vi "Global_ACT_Data Out.vi"() -> ()   [LabVIEW 2023, in "RingPlacer_ACT.lvlib"]
uses:
  startup.rtexe/RingPlacer_ACT.lvlib
  Cluster_Shooter Status.ctl
  startup.rtexe/Cluster_Speed Sensor Values.ctl
  startup.rtexe/Cluster_Velocity Values.ctl
  startup.rtexe/Cluster_Voltage Values.ctl
  startup.rtexe/Spark MAX Control Type.ctl
  startup.rtexe/Shooter_ACT.lvlib
panel:
  in  "ACT_RingPlacer_Control Mode":T1
  in  "ACT_RingPlacer_Status":T2
  in  "ACT_RingPlacer Motor Value":dbl
  in  "ACT_RingPlacer_CycleTime(S)":dbl
  # "The Names of the Data items in the Global Variable MUST describe who the Single Writer is\nFor Actuator Globals the the naming convention is\n   \nACT_Lib Name_Data Name\n\nExamples:\nACT_Drive_X axis\nACT_Hopper_AgitatorSpeed"
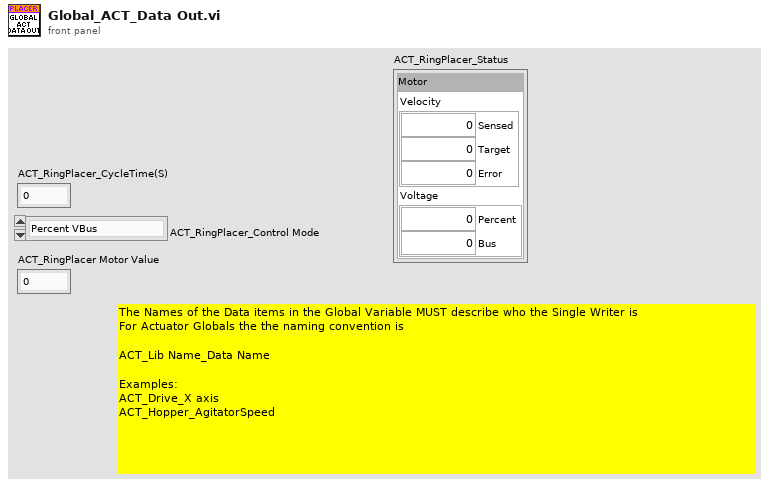
[diagram p1: front panel]
types:
  T1 = typedef "Spark MAX Control Type.ctl" = enum16{"Percent VBus", "Voltage", "Velocity", "Position", "Smart Motion", "Current", "Smart Velocity"}
  T2 = typedef "RingPlacer_ACT.lvlib/Cluster_Shooter Status.ctl" = cluster{"Motor":T3}
  T3 = typedef "Cluster_Speed Sensor Values.ctl" = cluster{"Velocity":T4, "Voltage":T5}
  T4 = typedef "Shooter_ACT.lvlib/Cluster_Velocity Values.ctl" = cluster{"Sensed":dbl, "Target":dbl, "Error":dbl}
  T5 = typedef "Shooter_ACT.lvlib/Cluster_Voltage Values.ctl" = cluster{"Percent":dbl, "Bus":dbl}
diagram:
